vi "Main.vi"() -> ()   [LabVIEW 2018]
uses:
  <vilib>/drjdpowell/SQLite Library/SQL Connection/Open (string).vi
  <vilib>/drjdpowell/SQLite Library/SQL Connection/Connection.lvclass
panel:
  in  "Tab Control":enum32{"Main", "Error"}(tab)
  in  "Path (txt. csv)":path
  in  "OK":bool
  in  "Button":bool
  in  "Table name":string
  in  "DB name":string
  out "error out":errorcluster
  out "Numeric":i32
  in  "error in":errorcluster
  in  "db exitst?":bool
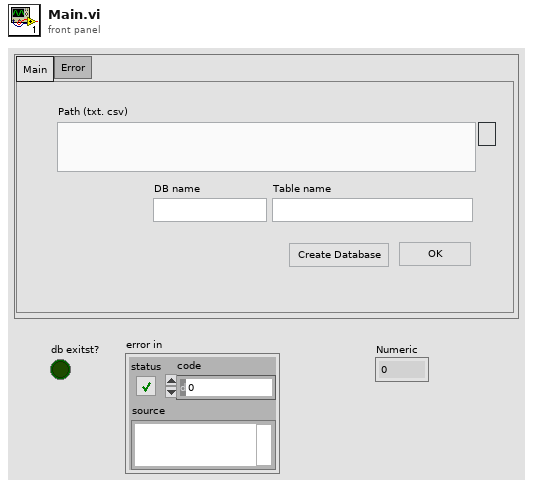
[diagram p1: front panel]
types:
  T1 = enum32{"Invalid", "Standard", "Closed", "Hidden", "Minimized", "Maximized"}
  T2 = enum32{"invalid app kind", "Development System", "Run Time System", "Student Edition", "Embedded LabVIEW", "Evaluation", "Custom"}
  T3 = enum8{"Enabled", "Disabled", "Disabled and Grayed Out"}
  T4 = enum16{"New or existing", "Existing", "Read only"}
  T5 = cluster{"Core":cluster{"Current VI Reference":refnum<vi>, "Close Panel on Exit?":bool}, "Date":string, "Table name":string, "Table Schema":string, "Table Elements":string, "ValsToInsert":string, "delimiter ":string, "File path":path, "File Extension ":string, "DB exist?":bool, "DB name ":string, "User name ":string}
  T6 = cluster{"Current VI Reference":refnum<vi>, "Close Panel on Exit?":bool}
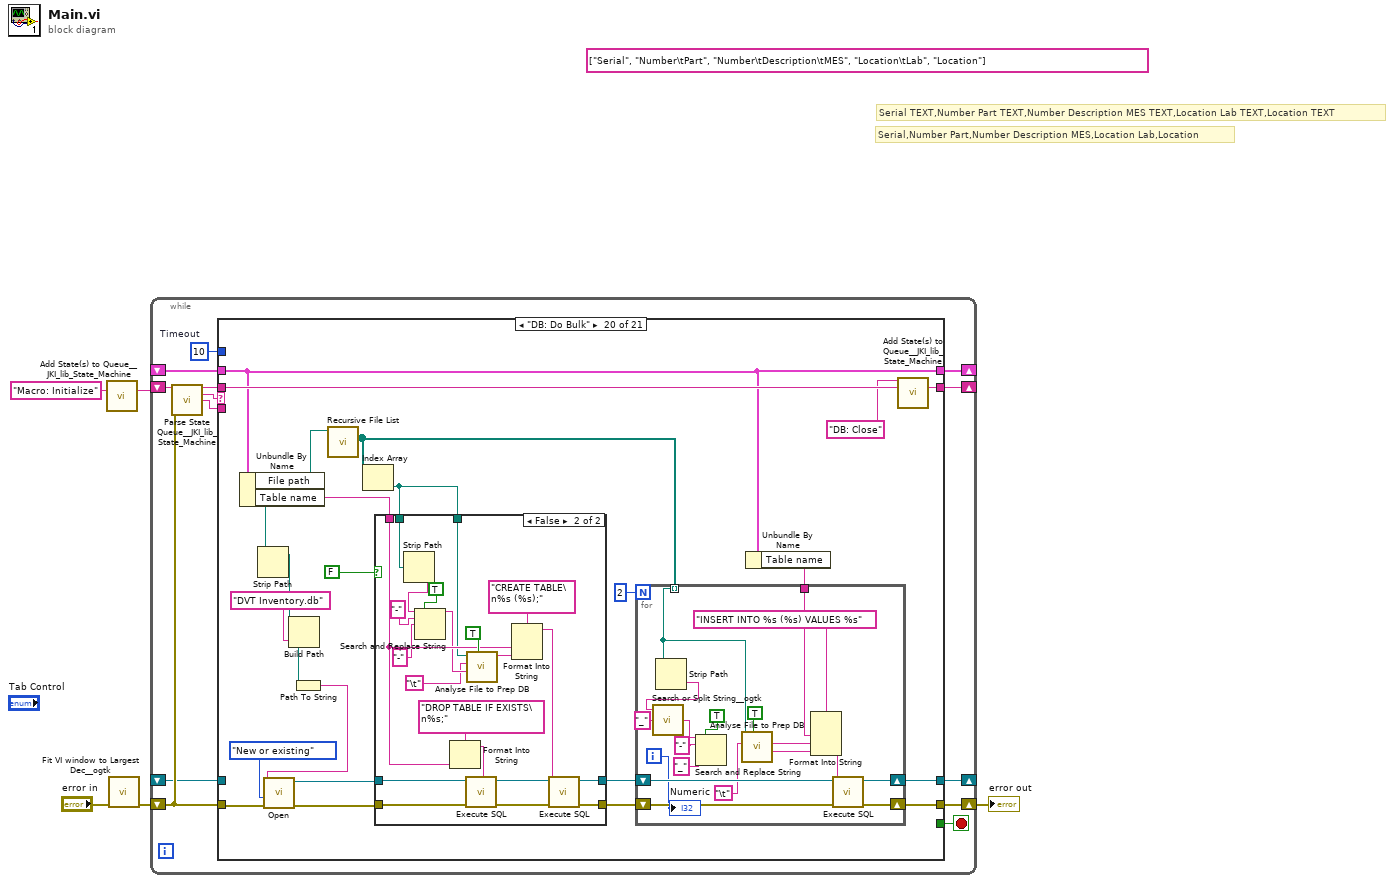
[diagram p0: block diagram]
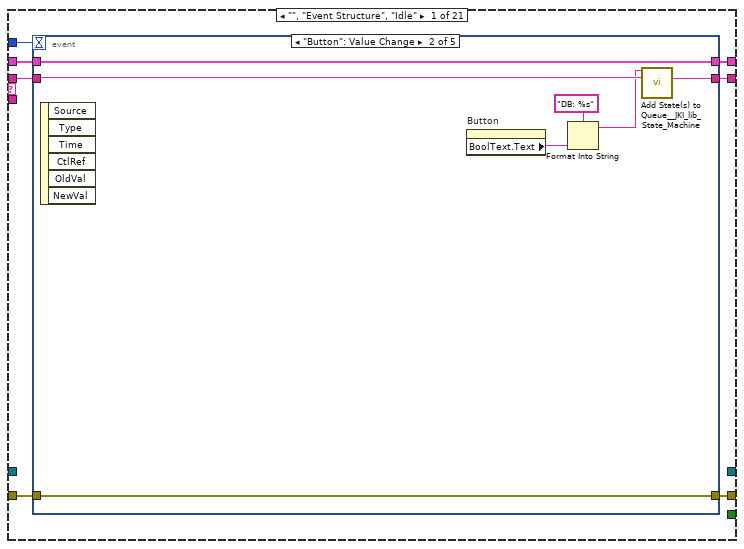
[diagram p2: hidden frame]
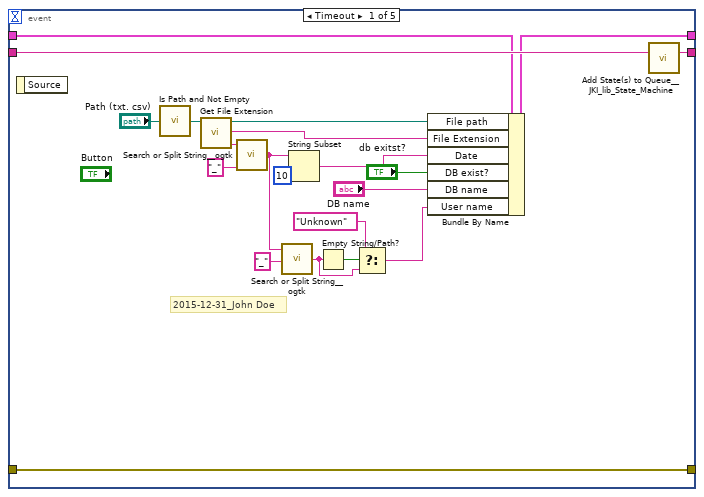
[diagram p3: hidden frame]
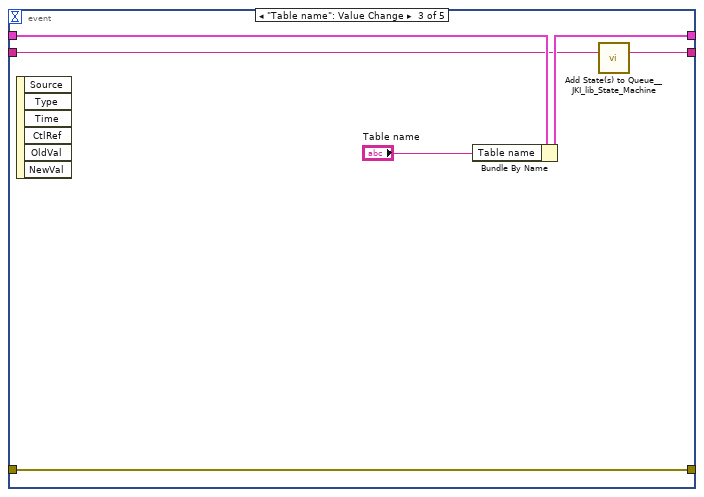
[diagram p4: hidden frame]
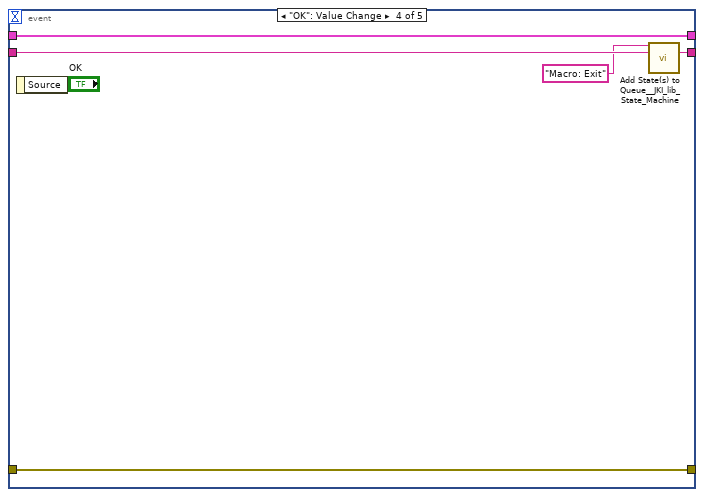
[diagram p5: hidden frame]
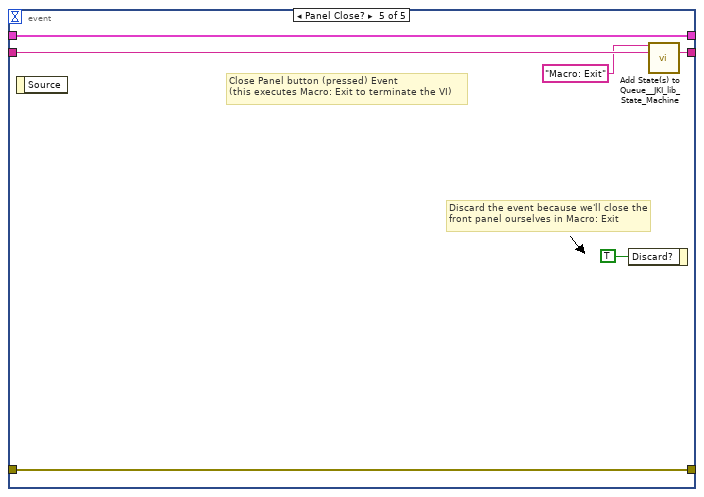
[diagram p6: hidden frame]
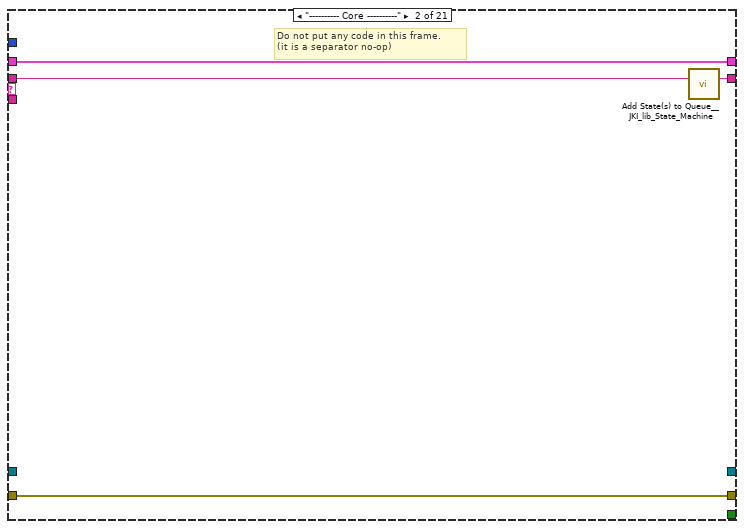
[diagram p7: hidden frame]
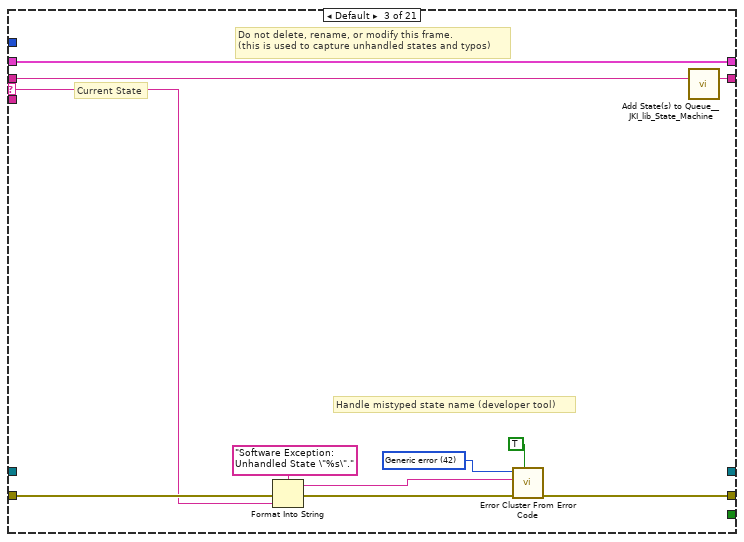
[diagram p8: hidden frame]
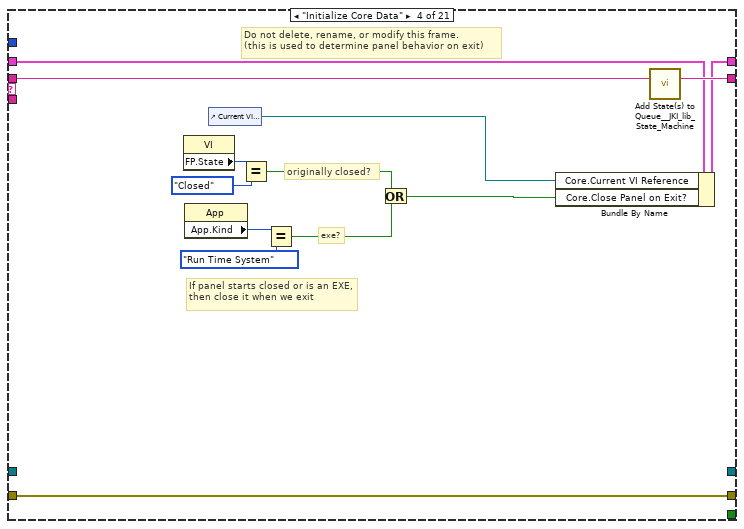
[diagram p9: hidden frame]
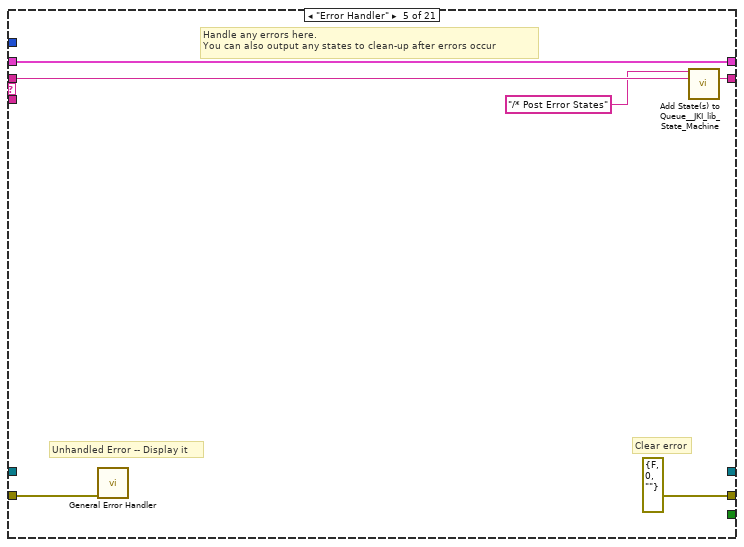
[diagram p10: hidden frame]
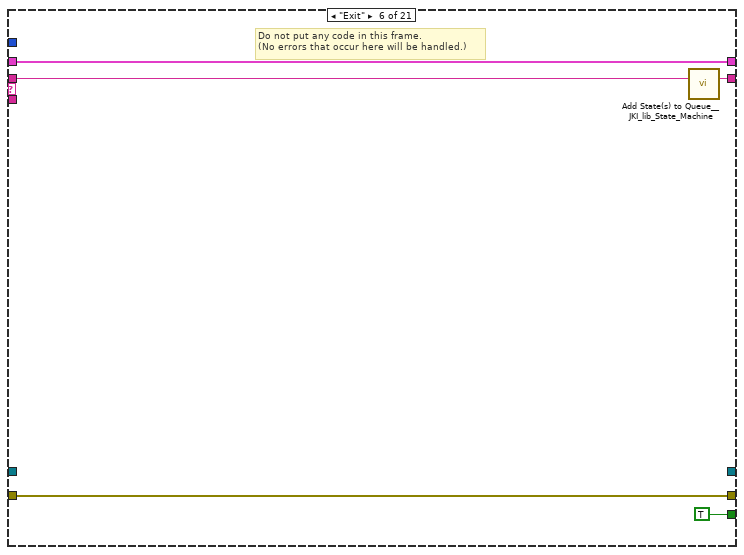
[diagram p11: hidden frame]
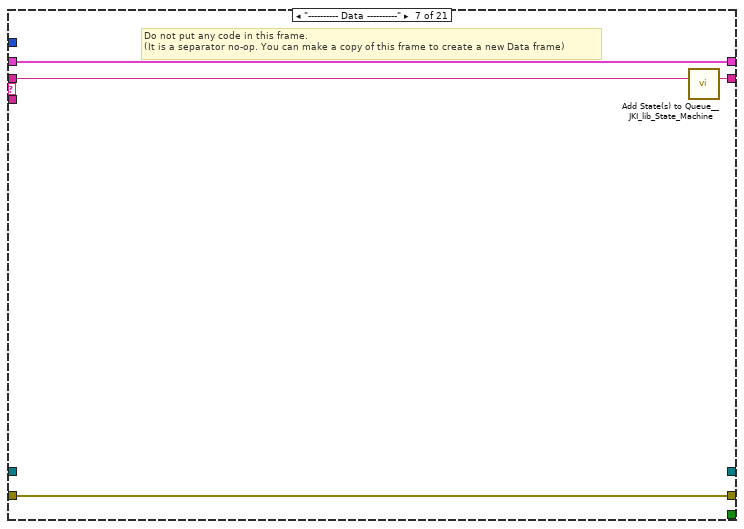
[diagram p12: hidden frame]
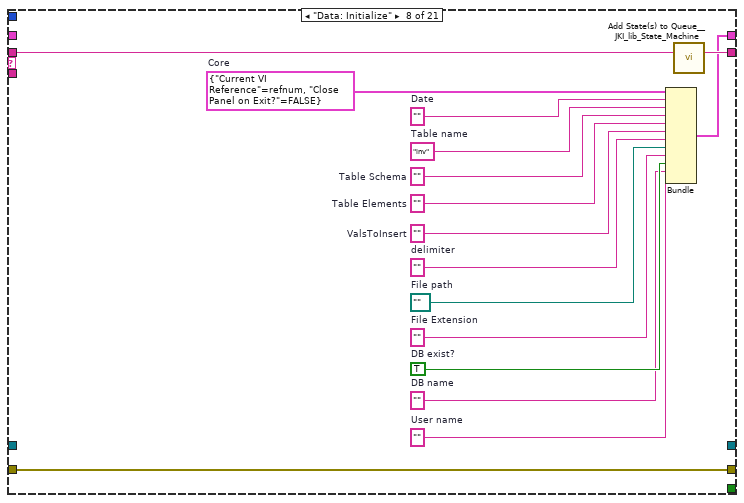
[diagram p13: hidden frame]
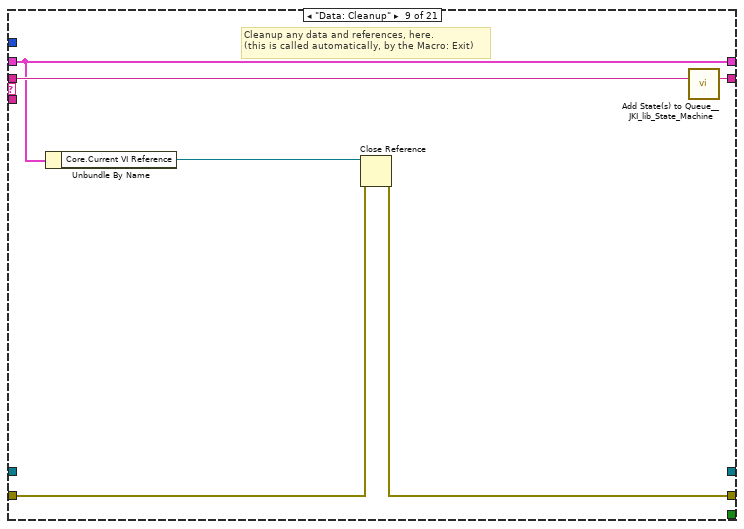
[diagram p14: hidden frame]
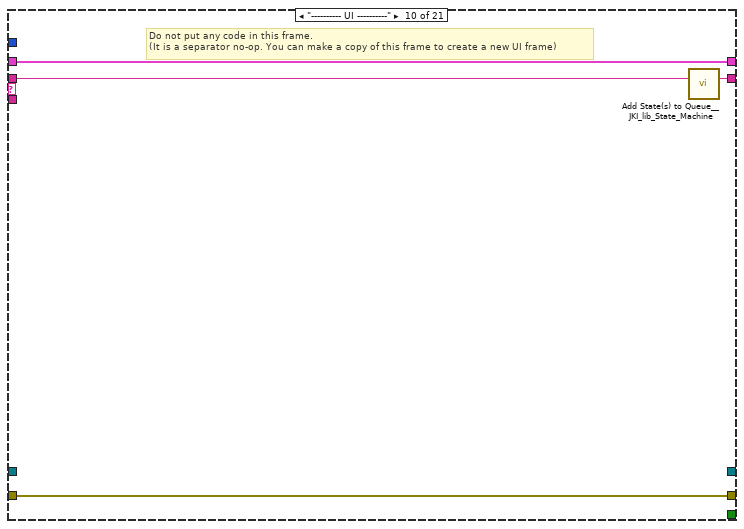
[diagram p15: hidden frame]
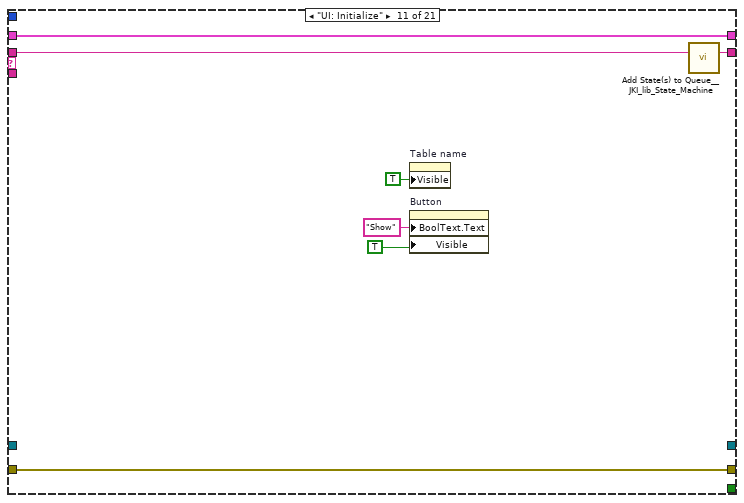
[diagram p16: hidden frame]
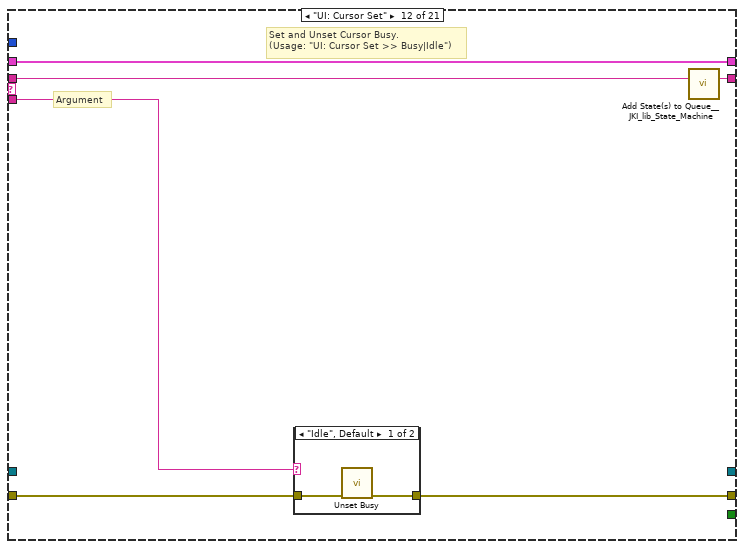
[diagram p17: hidden frame]
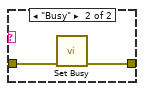
[diagram p18: hidden frame]
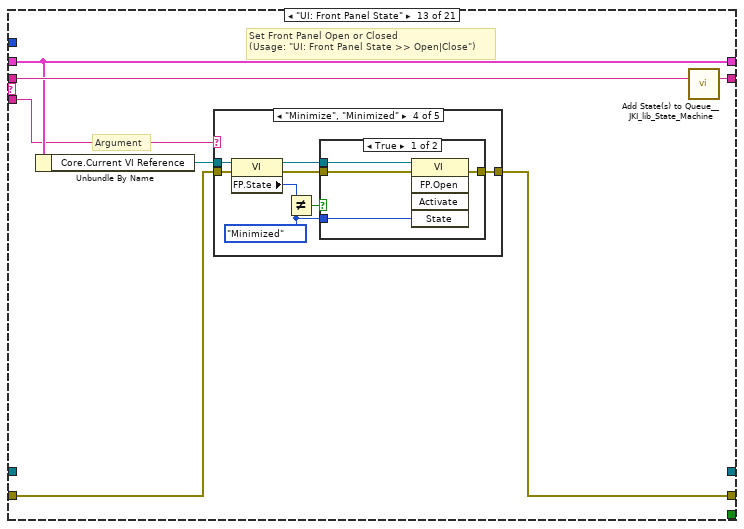
[diagram p19: hidden frame]
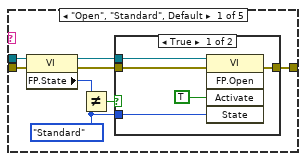
[diagram p20: hidden frame]
diagram:
  (unwired) string[] ["Serial", "Number\tPart", "Number\tDescription\tMES", "Location\tLab", "Location"] ("Header")
  # "Serial,Number\tPart,Number\tDescription\tMES,Location\tLab,Location"
  # "Serial TEXT,Number\tPart TEXT,Number\tDescription\tMES TEXT,Location\tLab TEXT,Location TEXT"
  n1 = call <vilib>:"Add State(s) to Queue__JKI_lib_State_Machine.vi"("State(s) in (\"\")"="Macro: Initialize") -> ("States Out"=w5:string)  [unwired: 14 in]
  n2 = call <userlib>:"Fit VI window to Largest Dec__ogtk.vi"("error in (no error)"="error in") -> ("error out"=w1:errorcluster)  [unwired: 5 in, 1 out]
  n3 = while {
    shift-right: [w11] -> _
    shift-left: _ -> [w10]
    shift-right: [w14] -> w3
    shift-left: w1 -> [w8]
    shift-right: [w13] -> _
    shift-left: w5 -> [w15]
    shift-right: [w7] -> _
    shift-left: _ -> [w6]
    stop <- w12 stop-if-true
    w9 = 10  # Timeout
    n4 = call <vilib>:"Parse State Queue__JKI_lib_State_Machine.vi"("State Queue"=w15, "Error In (no error)"=w8) -> ("Remaining States"=w17:string, "Current State"=w18:string, "Arguments"=w16:string)  [unwired: 11 in]
    n5 = case shown="\"DB: Do Bulk\"" w18 {
      selector: w18 -> [_ _ w73 _ _ _ _ _ _ _ _ _ _ _ _ _ _ _ _ _ _]
      tunnel: w17 -> [w25 w72 w77 w96 w102 w107 w111 w127 w133 w137 w144 w150 w161 w230 w235 w245 w249 w270 w295 w334 w383]
      tunnel: w16 -> [_ _ _ _ _ _ _ _ _ _ _ w145 w155 _ _ _ _ _ _ _ _]
      tunnel: w10 -> [w23 w69 w75 w89 w99 w105 w108 _ w128 w134 w142 w148 w157 w227 w232 w242 w246 w267 w273 w315 w381]
      tunnel: [w22 w70 w79 w93 errorcluster {"status"=FALSE, "code"=0, "source"=""} ("error out") w104 w109 w124 w129 w135 w141 w146 w158 w228 w233 w243 w247 w261 w276 w325 w378] -> w14
      tunnel: w8 -> [w21 w70 w78 w93 w98 w104 w109 w124 w130 w135 w141 w147 w159 w228 w233 w243 w247 w259 w293 w330 w380]
      tunnel: [w24 w71 w76 w95 w101 w106 w110 w126 w132 w136 w143 w149 w160 w229 w234 w244 w248 w269 w294 w333 w382] -> w13
      tunnel: [_ _ _ _ _ TRUE _ _ _ _ _ _ _ _ _ _ _ _ _ _ _] -> w12
      tunnel: [w20 w69 w75 w94 w99 w105 w108 w125 w128 w134 w142 w148 w157 w227 w232 w242 w246 w266 w273 w315 w381] -> w11
      tunnel: w9 -> [w19 _ _ _ _ _ _ _ _ _ _ _ _ _ _ _ _ _ _ _ _]
      tunnel: [_ _ _ _ _ _ _ _ _ _ _ _ _ _ _ _ _ _ w275 w324 _] -> w7
      tunnel: w6 -> [_ _ _ _ _ _ _ _ _ _ _ _ _ _ _ _ _ _ _ _ w379]
      frame "", "Event Structure", "Idle" {
        n6 = event shown="[1] \"Button\": Value Change" {
          selector: _ -> [_ _ _ _ _]
          dyn-events: _ -> [_ _ _ _ _]
          timeout: w19 -> [_ _ _ _ _]
          tunnel: w25 -> [w44 w49 w52 w62 w68]
          tunnel: [w43 w50 w53 w61 w67] -> w24
          tunnel: w23 -> [w41 w51 w57 w59 w65]
          tunnel: [w42 w48 w55 w60 w66] -> w22
          tunnel: w21 -> [w42 w48 w55 w60 w66]
          tunnel: [w39 w51 w56 w59 w65] -> w20
          event Timeout {
            # "2015-12-31_John Doe"
            n7 = event-data() -> ()  [unwired: 1 in, 1 out]
            n8 = call <vilib>:"Is Path and Not Empty.vi"("path"="Path (txt. csv)") -> ()  [unwired: 4 in, 1 out]
            n9 = call <vilib>:"Get File Extension.vi"("file"="Path (txt. csv)") -> ("filename without extension"=w38:string, "lowercase file extension"=w40:string)  [unwired: 6 in, 3 out]
            n10 = call <userlib>:"Search or Split String__ogtk.vi"("search string/char (-)"="_", "string"=w38) -> ("substring after match"=w31:string)  [unwired: 1 in, 2 out]
            n11 = call <userlib>:"Search or Split String__ogtk.vi"("search string/char (-)"="_", "string"=w31) -> ("substring after match"=w28:string)  [unwired: 1 in, 2 out]
            n12 = String Subset(string=w31, length (rest)=10 ("length (rest)")) -> (substring=w32:string)  [unwired: 1 in]
            n13 = Empty String/Path?(string/path=w28) -> (empty?=w29:bool)
            n14 = Select(t="Unknown" ("search string/char (-)"), s=w29, f=w28) -> (s? t:f=w26:string)
            n15 = Bundle By Name(cluster=w41, "File path"="Path (txt. csv)", "File Extension"=w40, "Date"=w32, "DB exist?"="db exitst?", "DB name"="DB name", "User name"=w26) -> (w39:T5)
            n16 = call <vilib>:"Add State(s) to Queue__JKI_lib_State_Machine.vi"("State(s) in (\"\")"=w44) -> ("States Out"=w43:string)  [unwired: 14 in]
          }
          event "Button": Value Change {
            n17 = event-data() -> ()  [unwired: 1 in, 6 out]
            n18 = property on="Button" class="Bool"() -> ("BoolText.Text"=w47:string)  [unwired: 2 in, 2 out]
            n19 = Format Into String(format string="DB: %s", w47) -> (resulting string=w45:string)  [unwired: 2 in, 1 out]
            n20 = call <vilib>:"Add State(s) to Queue__JKI_lib_State_Machine.vi"("State(s) in Front (\"\")"=w45, "State(s) in (\"\")"=w49) -> ("States Out"=w50:string)  [unwired: 13 in]
          }
          event "Table name": Value Change {
            n21 = event-data() -> ()  [unwired: 1 in, 6 out]
            n22 = Bundle By Name(cluster=w57, "Table name"="Table name") -> (w56:T5)
            n23 = call <vilib>:"Add State(s) to Queue__JKI_lib_State_Machine.vi"("State(s) in (\"\")"=w52) -> ("States Out"=w53:string)  [unwired: 14 in]
          }
          event "OK": Value Change {
            n24 = event-data() -> ()  [unwired: 1 in, 1 out]
            n25 = call <vilib>:"Add State(s) to Queue__JKI_lib_State_Machine.vi"("State(s) in Front (\"\")"="Macro: Exit", "State(s) in (\"\")"=w62) -> ("States Out"=w61:string)  [unwired: 13 in]
          }
          event Panel Close? {
            # "Discard the event because we'll close the front panel ourselves in Macro: Exit"
            # "Close Panel button (pressed) Event\n(this executes Macro: Exit to terminate the VI)"
            n26 = event-data() -> ()  [unwired: 1 in, 1 out]
            n27 = event-data("Discard?"=TRUE) -> ()  [unwired: 1 in, 1 out]
            n28 = call <vilib>:"Add State(s) to Queue__JKI_lib_State_Machine.vi"("State(s) in Front (\"\")"="Macro: Exit", "State(s) in (\"\")"=w68) -> ("States Out"=w67:string)  [unwired: 13 in]
          }
        }
      }
      frame "---------- Core ----------" {
        # "Do not put any code in this frame.\n(it is a separator no-op)"
        n29 = call <vilib>:"Add State(s) to Queue__JKI_lib_State_Machine.vi"("State(s) in (\"\")"=w72) -> ("States Out"=w71:string)  [unwired: 14 in]
      }
      frame Default {
        w82 = 42 items=["No error", "Argument error", "Memory is full", "Out of zone", "End of file", "File already open", "Generic file I/O error", "File not found", "File permission error", "Disk is full", "Duplicate path", "Too many files open", "System feature not enabled", "Resource file not found", "Cannot add resource", "Resource not found", "Image not found", "Image memory error", "Pen does not exist", "Config type invalid", "Config token not found", "Config parse error", "Config memory error", "Bad external code format", "Bad external code offset", "External code not present", "Null window", "Destroy window error", "Null menu", "Print aborted", "Bad print record", "Print driver error", "Windows error during printing", "Memory error during printing", "Print dialog error", "Generic print error", "Invalid device refnum", "Device not found", "Device parameter error", "Device unit error", "Cannot open device", "Device call aborted", "Generic error", "Cancelled by user", "Object ID too low", "Object ID too high", "Object not in heap", "Unknown heap", "Unknown object (invalid DefProc)", "Unknown object (DefProc not in table)", "Message out of range", "Invalid (null) method", "Unknown message", "Manager call not supported", "Bad address", "Network operation in progress", "Network operation timed out", "Connection is busy", "Network attribute not supported", "Network error", "Address in use", "System out of memory", "Connection aborted", "Connection refused", "Not connected", "Already connected", "Connection closed", "Initialization error (interapplication manager)", "Bad occurrence", "Wait on unbound occurrence handler", "Occurrence queue overflow", "Datalog type conflict", "Unused", "Unrecognized type (interapplication manager)", "Memory corrupt", "Failed to make temporary DLL", "Old CIN version", "Drag socket not found", "Failed to load drop-object", "Failed to register OLE object", "Failed to release OLE object", "Format specifier type mismatch", "Unknown format specifier", "Too few format specifiers", "Too many format specifiers", "Scan failed", "Newer CIN version", "Error converting to variant", "Runtime menu error", "Password tampered", "Variant attribute not found", "Incompatible variant data type", "Event data is not available", "Event Store is not present", "Occurrence is not found", "Event Queue is not created", "Event info is not available", "Refnum passed is NULL", "Error retrieving Class GUID", "Error retrieving CoClass GUID", "Error retrieving TypeLib GUID.", "Bad built application magic bytes.", "Specific driver is different from the specific driver associated with the Logical Name.", "There is no session opened to the class driver.", "Max Error", "MAX - Error with config objects", "MAX - Error loading configuration", "MAX - Group not supported"]
        # "Current State"
        # "Do not delete, rename, or modify this frame.\n(this is used to capture unhandled states and typos)"
        # "Handle mistyped state name (developer tool)"
        n30 = Format Into String(format string="Software Exception: Unhandled State \"%s\"." ("message"), error in=w78, w73) -> (resulting string=w81:string, error out=w80:errorcluster)  [unwired: 1 in]
        n31 = call <vilib>:"Error Cluster From Error Code.vi"("show call chain? (False)"=TRUE, "error in (no error)"=w80, "error message (\"\")"=w81, "error code (0)"=w82) -> ("error out"=w79:errorcluster)  [unwired: 5 in]
        n32 = call <vilib>:"Add State(s) to Queue__JKI_lib_State_Machine.vi"("State(s) in (\"\")"=w77) -> ("States Out"=w76:string)  [unwired: 14 in]
      }
      frame "Initialize Core Data" {
        # "Do not delete, rename, or modify this frame.\n(this is used to determine panel behavior on exit)"
        # "originally closed?"
        # "exe?"
        # "If panel starts closed or is an EXE, then close it when we exit"
        n33 = property class="VI"() -> ("FP.State"=w86:T1)  [unwired: 2 in, 2 out]
        n34 = property class="App"() -> ("App.Kind"=w92:T2)  [unwired: 2 in, 2 out]
        n35 = control-ref of="Current VI Reference"() -> (w87:refnum<vi>)
        n36 = Equal?(x=w86, y=T1."Closed" ("Front Panel Window:State")) -> (x = y?=w84:bool)
        n37 = Equal?(x=w92, y=T2."Run Time System" ("Application:Kind")) -> (x = y?=w90:bool)
        n38 = Or(x=w84, y=w90) -> (x .or. y?=w88:bool)
        n39 = Bundle By Name(cluster=w89, "Core.Current VI Reference"=w87, "Core.Close Panel on Exit?"=w88) -> (w94:T5)
        n40 = call <vilib>:"Add State(s) to Queue__JKI_lib_State_Machine.vi"("State(s) in (\"\")"=w96) -> ("States Out"=w95:string)  [unwired: 14 in]
      }
      frame "Error Handler" {
        # "Unhandled Error -- Display it"
        # "Handle any errors here.\nYou can also output any states to clean-up after errors occur"
        # "Clear error"
        n41 = call <vilib>:"General Error Handler.vi"("error in (no error)"=w98) -> ()  [unwired: 10 in, 5 out]
        n42 = call <vilib>:"Add State(s) to Queue__JKI_lib_State_Machine.vi"("State(s) in Front (\"\")"="/* Post Error States", "State(s) in (\"\")"=w102) -> ("States Out"=w101:string)  [unwired: 13 in]
      }
      frame "Exit" {
        # "Do not put any code in this frame.\n(No errors that occur here will be handled.)"
        n43 = call <vilib>:"Add State(s) to Queue__JKI_lib_State_Machine.vi"("State(s) in (\"\")"=w107) -> ("States Out"=w106:string)  [unwired: 14 in]
      }
      frame "---------- Data ----------" {
        # "Do not put any code in this frame.\n(It is a separator no-op. You can make a copy of this frame to create a new Data frame)"
        n44 = call <vilib>:"Add State(s) to Queue__JKI_lib_State_Machine.vi"("State(s) in (\"\")"=w111) -> ("States Out"=w110:string)  [unwired: 14 in]
      }
      frame "Data: Initialize" {
        w112 = ""  # User name
        w113 = ""  # DB name
        w114 = TRUE  # DB exist?
        w115 = ""  # File Extension
        w116 = path ""  # File path
        w117 = ""  # delimiter
        w118 = ""  # ValsToInsert
        w119 = ""  # Table Elements
        w120 = ""  # Table Schema
        w121 = "inv"  # Table name
        w122 = ""  # Date
        w123 = T6 {"Current VI Reference"=refnum, "Close Panel on Exit?"=FALSE}  # Core
        n45 = Bundle("Core"=w123, "Date"=w122, "Table name"=w121, "Table Schema"=w120, "Table Elements"=w119, "ValsToInsert"=w118, "delimiter"=w117, "File path"=w116, "File Extension"=w115, "DB exist?"=w114, "DB name"=w113, "User name"=w112) -> (w125:T5)  [unwired: 1 in]
        n46 = call <vilib>:"Add State(s) to Queue__JKI_lib_State_Machine.vi"("State(s) in (\"\")"=w127) -> ("States Out"=w126:string)  [unwired: 14 in]
      }
      frame "Data: Cleanup" {
        # "Cleanup any data and references, here.\n(this is called automatically, by the Macro: Exit)"
        n47 = Unbundle By Name(w128) -> ("Core.Current VI Reference"=w131:refnum<vi>)
        n48 = Close Reference(reference=w131, error in (no error)=w130) -> (error out=w129:errorcluster)
        n49 = call <vilib>:"Add State(s) to Queue__JKI_lib_State_Machine.vi"("State(s) in (\"\")"=w133) -> ("States Out"=w132:string)  [unwired: 14 in]
      }
      frame "---------- UI ----------" {
        # "Do not put any code in this frame.\n(It is a separator no-op. You can make a copy of this frame to create a new UI frame)"
        n50 = call <vilib>:"Add State(s) to Queue__JKI_lib_State_Machine.vi"("State(s) in (\"\")"=w137) -> ("States Out"=w136:string)  [unwired: 14 in]
      }
      frame "UI: Initialize" {
        n51 = property on="Table name" class="Str"("Visible"=TRUE) -> ()  [unwired: 2 in, 2 out]
        n52 = property on="Button" class="Bool"("BoolText.Text"="Show" ("Boolean Text.Text"), "Visible"=TRUE) -> ()  [unwired: 2 in, 2 out]
        n53 = call <vilib>:"Add State(s) to Queue__JKI_lib_State_Machine.vi"("State(s) in (\"\")"=w144) -> ("States Out"=w143:string)  [unwired: 14 in]
      }
      frame "UI: Cursor Set" {
        # "Argument"
        # "Set and Unset Cursor Busy.\n(Usage: \"UI: Cursor Set >> Busy|Idle\")"
        n54 = case shown="\"Idle\", Default" w145 {
          tunnel: w147 -> [w152 w154]
          tunnel: [w151 w153] -> w146
          frame "Idle", Default {
            n55 = call <vilib>:"Unset Busy.vi"("error in (no error)"=w152) -> ("error out"=w151:errorcluster)  [unwired: 10 in]
          }
          frame "Busy" {
            n56 = call <vilib>:"Set Busy.vi"("error in (no error)"=w154) -> ("error out"=w153:errorcluster)  [unwired: 9 in, 1 out]
          }
        }
        n57 = call <vilib>:"Add State(s) to Queue__JKI_lib_State_Machine.vi"("State(s) in (\"\")"=w150) -> ("States Out"=w149:string)  [unwired: 14 in]
      }
      frame "UI: Front Panel State" {
        # "Argument"
        # "Set Front Panel Open or Closed\n(Usage: \"UI: Front Panel State >> Open|Close\")"
        n58 = Unbundle By Name(w157) -> ("Core.Current VI Reference"=w156:refnum<vi>)
        n59 = case shown="\"Minimize\", \"Minimized\"" w155 {
          tunnel: w159 -> [w167 w182 w193 w206 w219]
          tunnel: [w169 w183 w195 w208 w221] -> w158
          tunnel: w156 -> [w168 w180 w194 w207 w220]
          frame "Open", "Standard", Default {
            w162 = T1."Standard" ("State")
            n60 = property class="VI"(reference=w168, error in=w167) -> (reference out=w165:refnum<vi>, error out=w166:errorcluster, "FP.State"=w164:T1)
            n61 = Not Equal?(x=w164, y=w162) -> (x != y?=w163:bool)
            n62 = case shown="True" w163 {
              tunnel: [w173 w175] -> w169
              tunnel: w166 -> [w172 w175]
              tunnel: w165 -> [w171 _]
              tunnel: w162 -> [w170 _]
              frame True {
                n63 = invoke class="VI" method="FP.Open"(reference=w171, error in=w172, "Activate"=TRUE, "State"=w170) -> (error out=w173:errorcluster)  [unwired: 1 in, 4 out]
              }
              frame False {
              }
            }
          }
          frame "Close", "Closed" {
            n64 = property class="VI"(reference=w180, error in=w182) -> (reference out=w179:refnum<vi>, error out=w181:errorcluster, "FP.State"=w177:T1)
            n65 = Not Equal?(x=w177, y=T1."Closed" ("Front Panel Window:State")) -> (x != y?=w176:bool)
            n66 = case shown="True" w176 {
              tunnel: [w184 w187] -> w183
              tunnel: w181 -> [w184 w186]
              tunnel: w179 -> [_ w185]
              frame False {
              }
              frame True {
                n67 = invoke class="VI" method="FP.Close"(reference=w185, error in=w186) -> (error out=w187:errorcluster)  [unwired: 1 in, 2 out]
              }
            }
          }
          frame "Hidden", "Hide" {
            w188 = T1."Hidden" ("State")
            n68 = property class="VI"(reference=w194, error in=w193) -> (reference out=w191:refnum<vi>, error out=w192:errorcluster, "FP.State"=w190:T1)
            n69 = Not Equal?(x=w190, y=w188) -> (x != y?=w189:bool)
            n70 = case shown="True" w189 {
              tunnel: [w199 w200] -> w195
              tunnel: w192 -> [w198 w200]
              tunnel: w191 -> [w197 _]
              tunnel: w188 -> [w196 _]
              frame True {
                n71 = invoke class="VI" method="FP.Open"(reference=w197, error in=w198, "State"=w196) -> (error out=w199:errorcluster)  [unwired: 2 in, 4 out]
              }
              frame False {
              }
            }
          }
          frame "Minimize", "Minimized" {
            w201 = T1."Minimized" ("State")
            n72 = property class="VI"(reference=w207, error in=w206) -> (reference out=w204:refnum<vi>, error out=w205:errorcluster, "FP.State"=w203:T1)
            n73 = Not Equal?(x=w203, y=w201) -> (x != y?=w202:bool)
            n74 = case shown="True" w202 {
              tunnel: [w212 w213] -> w208
              tunnel: w205 -> [w211 w213]
              tunnel: w204 -> [w210 _]
              tunnel: w201 -> [w209 _]
              frame True {
                n75 = invoke class="VI" method="FP.Open"(reference=w210, error in=w211, "State"=w209) -> (error out=w212:errorcluster)  [unwired: 2 in, 4 out]
              }
              frame False {
              }
            }
          }
          frame "Maximize", "Maximized" {
            w214 = T1."Maximized" ("State")
            n76 = property class="VI"(reference=w220, error in=w219) -> (reference out=w217:refnum<vi>, error out=w218:errorcluster, "FP.State"=w216:T1)
            n77 = Not Equal?(x=w216, y=w214) -> (x != y?=w215:bool)
            n78 = case shown="True" w215 {
              tunnel: [w225 w226] -> w221
              tunnel: w218 -> [w224 w226]
              tunnel: w217 -> [w223 _]
              tunnel: w214 -> [w222 _]
              frame True {
                n79 = invoke class="VI" method="FP.Open"(reference=w223, error in=w224, "State"=w222) -> (error out=w225:errorcluster)  [unwired: 2 in, 4 out]
              }
              frame False {
              }
            }
          }
        }
        n80 = call <vilib>:"Add State(s) to Queue__JKI_lib_State_Machine.vi"("State(s) in (\"\")"=w161) -> ("States Out"=w160:string)  [unwired: 14 in]
      }
      frame "---------- Macro ----------" {
        # "Do not put any code in this frame.\n(It is a separator no-op. You can make a copy of this frame to create a new Macro frame)"
        n81 = call <vilib>:"Add State(s) to Queue__JKI_lib_State_Machine.vi"("State(s) in (\"\")"=w230) -> ("States Out"=w229:string)  [unwired: 14 in]
      }
      frame "Macro: Initialize" {
        w231 = "Data: Initialize\nInitialize Core Data\nUI: Initialize\nUI: Front Panel State >> Open"  # Data: Initialize Initialize Core Data UI: Initialize UI: Front Panel State >> Open
        # "Initialization Macro\n(This is called once, when the VI starts)"
        n82 = call <vilib>:"Add State(s) to Queue__JKI_lib_State_Machine.vi"("State(s) in Front (\"\")"=w231, "State(s) in (\"\")"=w235) -> ("States Out"=w234:string)  [unwired: 13 in]
      }
      frame "Macro: Exit" {
        # "Exit Macro\n(This is called once, when the VI exits)"
        n83 = Unbundle By Name(w242) -> ("Core.Close Panel on Exit?"=w241:bool)
        n84 = Select(t="UI: Front Panel State >> Close", s=w241, f="") -> (s? t:f=w238:string)
        n85 = call <vilib>:"Add State(s) to Queue__JKI_lib_State_Machine.vi"("State(s) in (\"\")"=w238, "State(s) at Back (\"\")"="Data: Cleanup\nExit") -> ("States Out"=w236:string)  [unwired: 13 in]
        n86 = call <vilib>:"Add State(s) to Queue__JKI_lib_State_Machine.vi"("State(s) in Front (\"\")"=w236, "State(s) in (\"\")"=w245) -> ("States Out"=w244:string)  [unwired: 13 in]
      }
      frame "---------- New Category ----------" {
        # "Template Separator\n(You can make a copy of, or modify, this frame)"
        n87 = call <vilib>:"Add State(s) to Queue__JKI_lib_State_Machine.vi"("State(s) in (\"\")"=w249) -> ("States Out"=w248:string)  [unwired: 14 in]
      }
      frame "DB: Show" {
        w252 = "-" ("search string")
        w257 = TRUE ("Visible")
        n88 = Unbundle By Name(w267) -> ("File path"=w268:path, "Date"=w256:string, "User name"=w251:string)
        n89 = Search and Replace String(replace all?=TRUE ("replace all? (F)"), input string=w256, search string=w252, replace string=w252) -> (result string=w255:string)  [unwired: 4 in, 3 out]
        n90 = call "Analyse File to Prep DB.vi"("Dummy Data 2"=w251, "Dummy fill?"=FALSE, "error in (no error)"=w259, "Dummy Data"=w255, "Delimiter"=",", "Txt  file"=w268) -> ("error out"=w262:errorcluster, "Value to be inserted"=w263:string, "Table Elements"=w264:string, "Table Schema"=w265:string)  [unwired: 2 in]
        n91 = Bundle By Name(cluster=w267, "Table Schema"=w265, "Table Elements"=w264, "ValsToInsert"=w263) -> (w266:T5)
        n92 = property on="Button" class="Bool"(error in=w262, "BoolText.Text"="CreateDatabBase" ("Boolean Text.Text"), "DisabledEnum"=T3."Enabled" ("Disabled")) -> (error out=w261:errorcluster)  [unwired: 1 in, 1 out]
        n93 = property on="Table name" class="Str"("Visible"=w257, "Key Focus"=w257) -> ()  [unwired: 2 in, 2 out]
        n94 = call <vilib>:"Add State(s) to Queue__JKI_lib_State_Machine.vi"("State(s) in (\"\")"=w270) -> ("States Out"=w269:string)  [unwired: 14 in]
      }
      frame "DB: CreateDatabBase" {
        n95 = Unbundle By Name(w273) -> ("DB exist?"=w272:bool, "File path"=w281:path, "DB name"=w271:string)
        n96 = Strip Path(path=w281) -> (stripped path=w282:path)  [unwired: 1 out]
        n97 = Format Into String(format string="%s.db", w271) -> (resulting string=w279:string)  [unwired: 2 in, 1 out]
        n98 = Build Path(base path=w282, name or relative path=w279) -> (appended path=w278:path)
        n99 = Path To String(path=w278) -> (string=w277:string)
        n100 = call-poly <vilib>:"Open.vi"("error in (no error)"=w293, "File Option"=T4."New or existing", "db file"=w277) -> ("error out"=w291:errorcluster, "SQLite Connection out"=w292:refnum<class "Connection.lvclass">)  [unwired: 7 in]
        n101 = case shown="False" w272 {
          tunnel: w292 -> [w297 w311]
          tunnel: w291 -> [w296 w310]
          tunnel: [w296 w303] -> w290
          tunnel: [w297 w302] -> w289
          tunnel: w273 -> [_ w301]
          frame True {
          }
          frame False {
            n102 = Unbundle By Name(w301) -> ("Table name"=w309:string, "Table Schema"=w308:string)
            n103 = Unbundle By Name(w301) -> ("Table name"=w298:string)
            n104 = Format Into String(format string="DROP TABLE IF EXISTS\n%s;", w298) -> (resulting string=w299:string)  [unwired: 2 in, 1 out]
            n105 = call <vilib>:"Execute SQL.vi"("error in (no error)"=w310, "SQL"=w299, "SQLite Connection in"=w311) -> ("error out"=w304:errorcluster, "SQLite Connection out"=w306:refnum<class "Connection.lvclass">)  [unwired: 5 in, 2 out]
            n106 = Format Into String(format string="CREATE TABLE\n%s (%s);", w309, w308) -> (resulting string=w305:string)  [unwired: 2 in, 1 out]
            n107 = call <vilib>:"Execute SQL.vi"("error in (no error)"=w304, "SQL"=w305, "SQLite Connection in"=w306) -> ("error out"=w303:errorcluster, "SQLite Connection out"=w302:refnum<class "Connection.lvclass">)  [unwired: 5 in, 2 out]
          }
        }
        n108 = Unbundle By Name(w273) -> ("Table name"=w287:string, "Table Elements"=w286:string, "ValsToInsert"=w285:string)
        n109 = Format Into String(format string="INSERT INTO %s (%s) VALUES %s", w287, w286, w285) -> (resulting string=w284:string)  [unwired: 2 in, 1 out]
        n110 = call <vilib>:"Execute SQL.vi"("error in (no error)"=w290, "SQL"=w284, "SQLite Connection in"=w289) -> ("error out"=w276:errorcluster, "SQLite Connection out"=w275:refnum<class "Connection.lvclass">)  [unwired: 5 in, 2 out]
        n111 = call <vilib>:"Add State(s) to Queue__JKI_lib_State_Machine.vi"("State(s) in Front (\"\")"="DB: Close" ("State(s) in Front (\"\")"), "State(s) in (\"\")"=w295) -> ("States Out"=w294:string)  [unwired: 13 in]
      }
      frame "DB: Do Bulk" {
        n112 = Unbundle By Name(w315) -> ("File path"=w322:path, "Table name"=w316:string)
        n113 = Strip Path(path=w322) -> (stripped path=w321:path)  [unwired: 1 out]
        n114 = Build Path(base path=w321, name or relative path="DVT Inventory.db") -> (appended path=w319:path)
        n115 = Path To String(path=w319) -> (string=w318:string)
        n116 = call-poly <vilib>:"Open.vi"("error in (no error)"=w330, "File Option"=T4."New or existing", "db file"=w318) -> ("error out"=w329:errorcluster, "SQLite Connection out"=w328:refnum<class "Connection.lvclass">)  [unwired: 7 in]
        n117 = call <vilib>:"Recursive File List.vi"("Folder Path"=w322) -> ("All Files in Dir"=w317:path[])  [unwired: 6 in, 4 out]
        n118 = Index Array(array=w317) -> (element=w313:path)  [unwired: 1 in]
        n119 = case shown="False" FALSE {
          tunnel: w328 -> [w355 w368]
          tunnel: w329 -> [w354 w367]
          tunnel: [w354 w372] -> w326
          tunnel: [w355 w371] -> w327
          tunnel: w313 -> [_ w363]
          tunnel: w316 -> [_ w364]
          tunnel: w313 -> [_ w362]
          frame True {
          }
          frame False {
            n120 = Strip Path(path=w362) -> (name=w360:string)  [unwired: 1 out]
            n121 = Search and Replace String(replace all?=TRUE ("replace all? (F)"), input string=w360, search string="-", replace string="-" ("search string")) -> (result string=w357:string)  [unwired: 4 in, 3 out]
            n122 = Format Into String(format string="DROP TABLE IF EXISTS\n%s;", w364) -> (resulting string=w369:string)  [unwired: 2 in, 1 out]
            n123 = call <vilib>:"Execute SQL.vi"("error in (no error)"=w367, "SQL"=w369, "SQLite Connection in"=w368) -> ("error out"=w373:errorcluster, "SQLite Connection out"=w375:refnum<class "Connection.lvclass">)  [unwired: 5 in, 2 out]
            n124 = call "Analyse File to Prep DB.vi"("Dummy fill?"=TRUE, "Dummy Data"=w357, "Delimiter"="\t", "Txt  file"=w363) -> ("Table Schema"=w366:string)  [unwired: 4 in, 3 out]
            n125 = Format Into String(format string="CREATE TABLE\n%s (%s);", w364, w366) -> (resulting string=w374:string)  [unwired: 2 in, 1 out]
            n126 = call <vilib>:"Execute SQL.vi"("error in (no error)"=w373, "SQL"=w374, "SQLite Connection in"=w375) -> ("error out"=w372:errorcluster, "SQLite Connection out"=w371:refnum<class "Connection.lvclass">)  [unwired: 5 in, 2 out]
          }
        }
        n127 = Unbundle By Name(w315) -> ("Table name"=w314:string)
        n128 = for {
          N: 2 -> [_]
          shift-right: [w343] -> w324
          shift-left: w327 -> [w348]
          shift-right: [w344] -> w325
          shift-left: w326 -> [w347]
          tunnel: w317 -> [w342] mode=indexing
          tunnel: w314 -> [w341]
          i -> [w338]
          n129 = Strip Path(path=w342) -> (name=w337:string)  [unwired: 1 out]
          n130 = call <userlib>:"Search or Split String__ogtk.vi"("search string/char (-)"="_", "string"=w337) -> ("substring after match"=w335:string)  [unwired: 1 in, 2 out]
          n131 = Search and Replace String(replace all?=TRUE ("replace all? (F)"), input string=w335, search string="-", replace string="_" ("search string")) -> ()  [unwired: 4 in, 4 out]
          n132 = call "Analyse File to Prep DB.vi"("Dummy fill?"=TRUE, "Delimiter"="\t", "Txt  file"=w342) -> ("Value to be inserted"=w346:string, "Table Elements"=w345:string)  [unwired: 5 in, 2 out]
          n133 = Format Into String(format string="INSERT INTO %s (%s) VALUES %s", w341, w345, w346) -> (resulting string=w349:string)  [unwired: 2 in, 1 out]
          n134 = call <vilib>:"Execute SQL.vi"("error in (no error)"=w347, "SQL"=w349, "SQLite Connection in"=w348) -> ("error out"=w344:errorcluster, "SQLite Connection out"=w343:refnum<class "Connection.lvclass">)  [unwired: 5 in, 2 out]
          "Numeric" <- w338
        }
        n135 = call <vilib>:"Add State(s) to Queue__JKI_lib_State_Machine.vi"("State(s) in Front (\"\")"="DB: Close" ("State(s) in Front (\"\")"), "State(s) in (\"\")"=w334) -> ("States Out"=w333:string)  [unwired: 13 in]
      }
      frame "DB: Close" {
        n136 = call-dynamic "Close.vi"("error in (no error)"=w380, "SQLite Connection in"=w379) -> ("error out"=w378:errorcluster)  [unwired: 9 in]
        n137 = call <vilib>:"Add State(s) to Queue__JKI_lib_State_Machine.vi"("State(s) in Front (\"\")"="Macro: Exit" ("State(s) in Front (\"\")"), "State(s) in (\"\")"=w383) -> ("States Out"=w382:string)  [unwired: 13 in]
      }
    }
  }
  "error out" <- w3
